vi "Read.PITCH.File.vi"(10 "Raw File":string="raw.pitch.dat", 11 "Path":path=path "E:/work/Arty/arty_bats/labview/Test") -> (3 "data":u8[](array[numeric]) format="%.0x")   [LabVIEW 2020]
panel:
  out "Hdr Length":u16
  out "Hdr Sequence":u32
  out "Hdr Unit":u8
  out "Hdr Count":u8
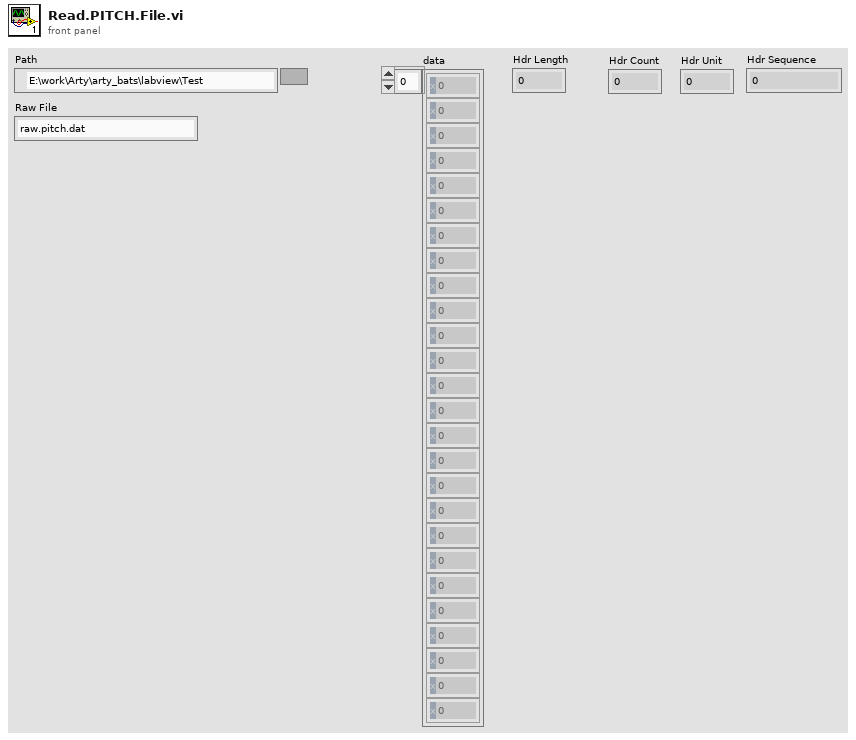
[diagram p1: front panel]
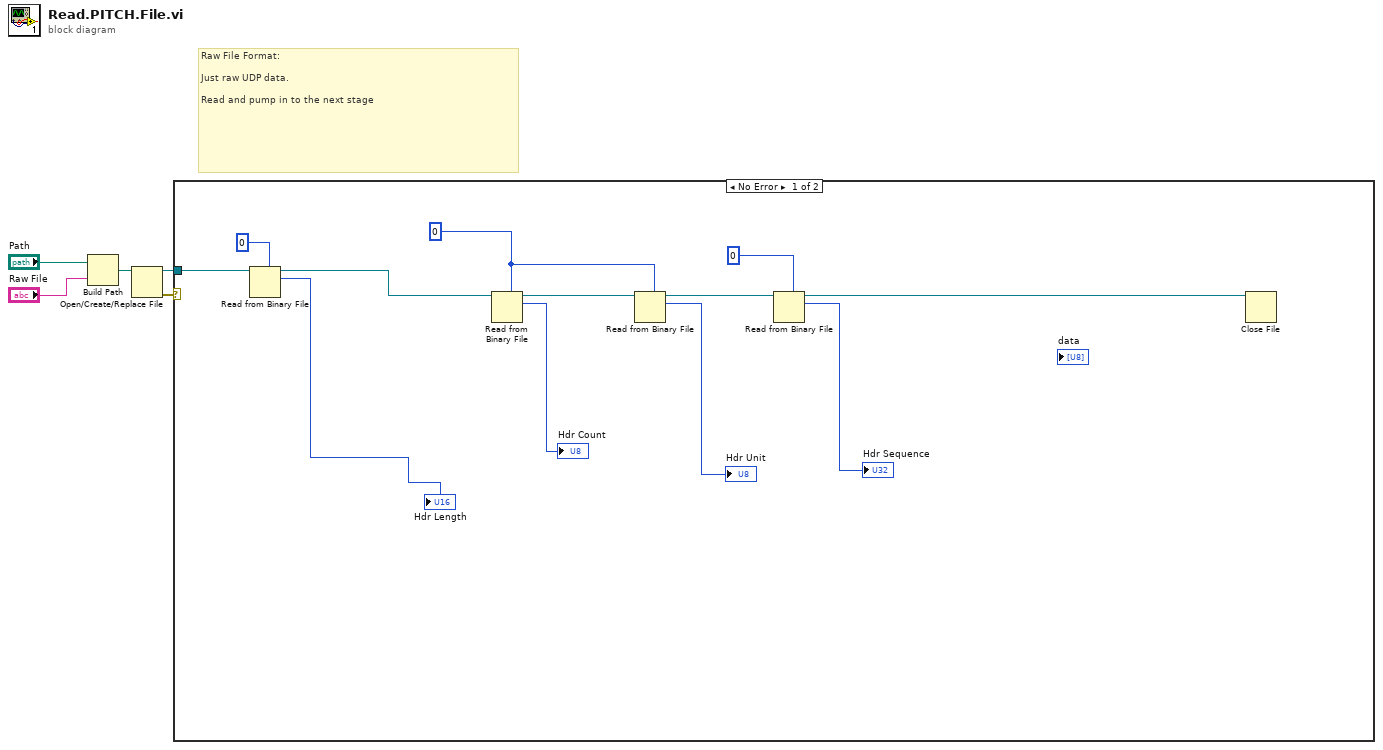
[diagram p0: block diagram]
diagram:
  # "Raw File Format:\n\nJust raw UDP data.\n\nRead and pump in to the next stage"
  n1 = Build Path(base path="Path", name or relative path="Raw File") -> (appended path=w3:path)
  n2 = Open/Create/Replace File(file path (use dialog)=w3) -> (refnum out=w1:refnum<file>, error out=w2:errorcluster)  [unwired: 5 in, 1 out]
  n3 = case shown="No Error" w2 {
    tunnel: w1 -> [w17 _]
    frame No Error {
      w9 = u8 0 ("count (1)")
      n4 = Read from Binary File(5:u16 0 ("count (1)"), 11:w17) -> (2:→"Hdr Length":u16, 3:w14:refnum<file>)  [unwired: 4 in, 2 out]
      n5 = Read from Binary File(5:w9, 11:w14) -> (2:→"Hdr Count":u8, 3:w12:refnum<file>)  [unwired: 4 in, 2 out]
      n6 = Read from Binary File(5:w9, 11:w12) -> (2:→"Hdr Unit":u8, 3:w11:refnum<file>)  [unwired: 4 in, 2 out]
      n7 = Read from Binary File(5:u32 0 ("count (1)"), 11:w11) -> (2:→"Hdr Sequence":u32, 3:w10:refnum<file>)  [unwired: 4 in, 2 out]
      n8 = Close File(refnum=w10) -> ()  [unwired: 1 in, 2 out]
    }
    frame Error {
    }
  }
